vi "poc.test.vi"() -> ()   [LabVIEW 2020]
uses:
  <vilib>/Platform/TimedLoop/XDataNode/timing_clust.ctl
  <vilib>/Platform/TimedLoop/XDataNode/nitl_modes.ctl
  <vilib>/Platform/TimedLoop/XDataNode/wakeup.ctl
  axi_2_eth_raw.ctl
  <vilib>/rvi/DataTransferAndStorage/Container/Common/niFpgaContainerGetUniqueNameForEmu.vi
  <vilib>/rvi/DataTransferAndStorage/Container/Common/niFpgaContainerSetEmuInfo.vi
  <vilib>/rvi/eio/common/nirviEmuReportErrorAndStop.vi
  <vilib>/rvi/Emulation/niFpgaSctlEmulationGetInTimedLoop.vi
  <vilib>/rvi/Emulation/niFpgaEmulationReportErrorSimple.vi
  <vilib>/rvi/Emulation/niFpgaGetClockAttributes.vi
  <vilib>/rvi/Emulation/niFpgaCriticalErrorInLSC.vi
  <vilib>/rvi/DataTransferAndStorage/Container/Common/niFpgaContainerExecOnDevCompGetState.vi
  <vilib>/rvi/Emulation/niFpgaEmulationIsFPGAContextNoSignature.vi
  <vilib>/rvi/errors/niFpgaSetErrorForExecOnDevCompSimple.vi
  <vilib>/rvi/FIFO/Fifo_Resource/nirvififoEmulationSetSize.vi
  <vilib>/rvi/FIFO/Fifo_Resource/nirviFifoEmulationQueueMgr.vi
  <instcachedir>/0/nirviFifoEmulationQueueMgr_E5CAEC123FF24DC58D834DCA3CDAA9B5.lvgen/nirviFifoEmulationQueueMgr_E5CAEC123FF24DC58D834DCA3CDAA9B5_018.vi
  <vilib>/rvi/FIFO/Fifo_Resource/nirvififoEmulationDetermineInputValidOut.vi
  <vilib>/rvi/FIFO/Fifo_Resource/nirvififoEmulationCreateLock.vi
  <vilib>/rvi/Emulation/niFpgaProcessEmulError.vi
  <vilib>/rvi/FIFO/Fifo_Resource/nirvififoEmulationObtainLock.vi
  <vilib>/rvi/FIFO/Fifo_Resource/nirvififoEmulationReleaseLock.vi
  <vilib>/rvi/occurrence/nirviWaitOnOccurrenceBase.vi
  <vilib>/rvi/errors/nirviReportUnexpectedCaseInternalError.vi
  <vilib>/rvi/errors/nirviReportUnexpectedCaseInternalError (U32).vi
  <vilib>/Utility/error.llb/Clear Errors.vi
  <vilib>/rvi/interface/RandomDataEmulation/niFpgaRandomDataHandleErrors.vi
  <instcachedir>/0/nirviFifoEmulationQueueMgr_E5CAEC123FF24DC58D834DCA3CDAA9B5.lvgen/nirviFifoEmulationQueueMgr_E5CAEC123FF24DC58D834DCA3CDAA9B5_020.vi
  <vilib>/rvi/interface/RandomDataEmulation/nirviRandomDataMultiElementFPGAFIFO.vi
  <instcachedir>/0/nirviRandomDataMultiElementFPGAFIFO_3E9965BA1FAD4E7B8DABA31768A09B1F.lvgen/nirviRandomDataMultiElementFPGAFIFO_3E9965BA1FAD4E7B8DABA31768A09B1F_001.vi
  <instcachedir>/0/nirviFifoEmulationQueueMgr_E5CAEC123FF24DC58D834DCA3CDAA9B5.lvgen/nirviFifoEmulationQueueMgr_E5CAEC123FF24DC58D834DCA3CDAA9B5_017.vi
  <vilib>/rvi/Memory/Memory_Emulation/niFpgaMemoryEmulationCacheClearOnFirstRun.vi
  <vilib>/rvi/Memory/Memory_Emulation/nirvimemoryEmulationManagerCache_MakeExclusive.vi
  <vilib>/rvi/Memory/Memory_Emulation/niFpgaMemoryEmulationValidateCache.vi
  <vilib>/rvi/Memory/Memory_Emulation/nirvimemoryEmulationManagerCache_InsertValue.vi
  <vilib>/rvi/Memory/Memory_Emulation/nirvimemoryEmulationManagerCache_ReleaseExclusive.vi
  <vilib>/rvi/Memory/Memory_Emulation/nirvimemoryEmulationManagerCache_GetValue.vi
  <vilib>/rvi/Memory/Memory_Emulation/nirvimemoryEmulationManagerCache_SetValue.vi
  <vilib>/rvi/Emulation/niFpgaSctlEmulationResourceMgr.vi
  <vilib>/Platform/TimedLoop/XDataNode/XDataNode.xnode
  <vilib>/rvi/LocalResourceManager/LocalResourceManager.xnode
  <vilib>/rvi/DataTransferAndStorage/Container/XNode/niFpgaContainer.xnode
  <vilib>/rvi/FIFO/Fifo_Resource/niFpgaFifoEmulationRefIn.vi
  <vilib>/rvi/FIFO/Fifo_Resource/nirvififoEmulationRead.vi
  <vilib>/rvi/interface/RandomDataEmulation/nirviRandomDataFpgaMultiElementTemplate.vi
  <vilib>/rvi/Memory/Memory_Emulation/niFpgaMemoryEmulationRefIn.vi
  <vilib>/Platform/TimedLoop/XDataNode/XDNodeRunTimeDep.lvlib
  submodules/Market.Data.Common/fpga/fpganow.common.fpga.lvlib
panel:
  in  "ip.Reset":bool
  out "i":u16
  out "Data":T1
  out "Numeric":i32
  in  "Reset":bool
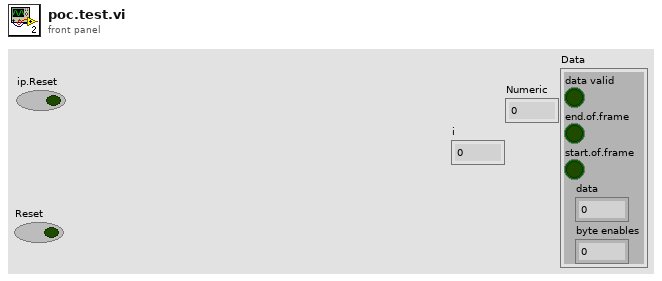
[diagram p1: front panel]
types:
  T1 = cluster{"data valid":bool, "end.of.frame":bool, "start.of.frame":bool, "data":u64, "byte enables":u8}
  T2 = typedef "XDNodeRunTimeDep.lvlib/timing_clust.ctl" = cluster{"Expected End [f-1]":u64, "Actual End [f-1]":u64, "Finished Late? [f-1]":bool, "Expected End [i-1]":u64, "Actual End [i-1]":u64, "Finished Late? [i-1]":bool, "Expected Start [i]":u64, "Actual Start [i]":u64, "Expected Start [f]":u64, "Actual Start [f]":u64, "Source Name":string, "Structure Name":string, "Period":i64, "Deadline":i64, "Offset":i64, "Start":i64, "Priority":i32, "Timeout":i32, "Mode":T3, "Wakeup Reason":T4, "Error":errorcluster, "Source Type":string, "Secondary Source Type":string, "Global End Time":u64, "Global Start Time":u64, "Frame Duration":u64, "Iteration Duration":u64, "Assigned CPU":i32, "I/O Scan Engine Mode":u32}
  T3 = typedef "XDNodeRunTimeDep.lvlib/nitl_modes.ctl" = enum32{"No Change", "Process missed periods, maintain original phase", "Discard missed periods, maintain original phase", "Process missed periods, ignore original phase", "Discard missed periods, ignore original phase"}
  T4 = typedef "XDNodeRunTimeDep.lvlib/wakeup.ctl" = enum32{"Normal", "Aborted", "Asynchronous wakeup", "Timing source error", "Timed loop error", "Timeout"}
  T5 = typedef "axi_2_eth_raw.ctl" = cluster{"data valid":bool, "end.of.frame":bool, "start.of.frame":bool, "data":u64, "byte enables":u8}
  T6 = cluster{"type":enum8{"Time", "AddOrder", "OrderExecuted", "OrderExecutedAtPrice", "ReduceSize", "ModifyOrder", "DeleteOrder", "Get.Everything", "Get.All.Orders", "Get.Top"}, "side":u8, "orderId ":u64, "quantity":u32, "symbol":u64, "price":u64, "executed.qty":u32, "canceled.qty":u32, "remaining.qty":u32, "seconds":u64, "nanoseconds":u64, "Add":bool, "Edit":bool, "Remove":bool, "seq no":u32, "recv.time":u64, "parse.time":u64}
  T7 = enum8{"Time", "AddOrder", "OrderExecuted", "OrderExecutedAtPrice", "ReduceSize", "ModifyOrder", "DeleteOrder", "Get.Everything", "Get.All.Orders", "Get.Top"}
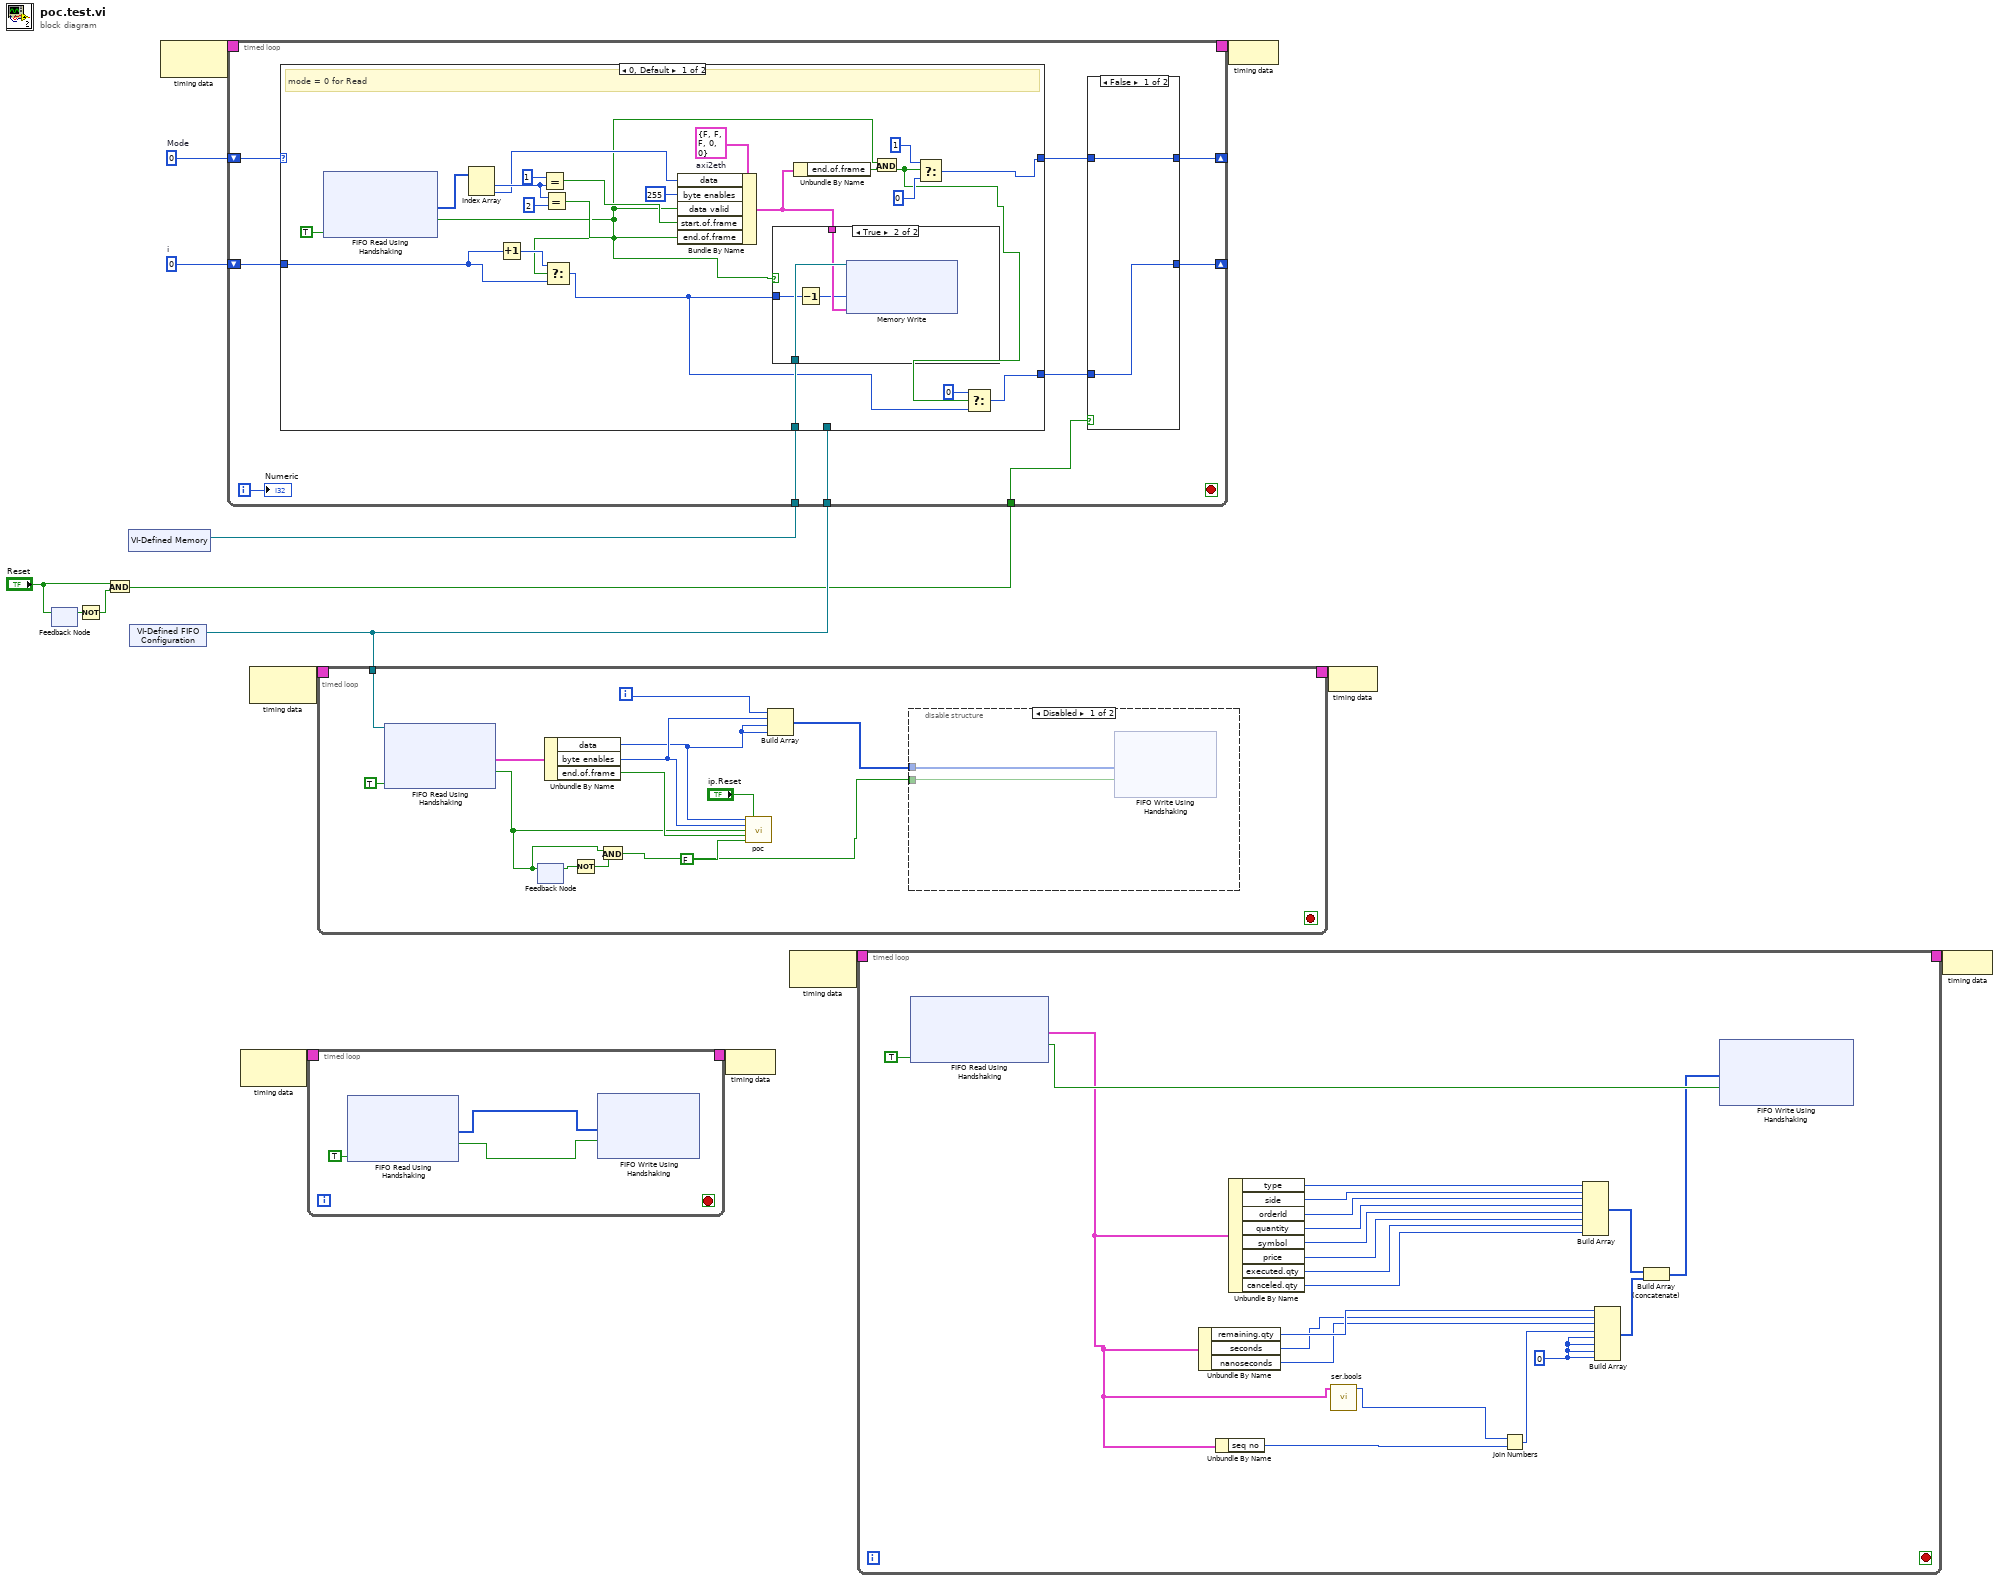
[diagram p0: block diagram]
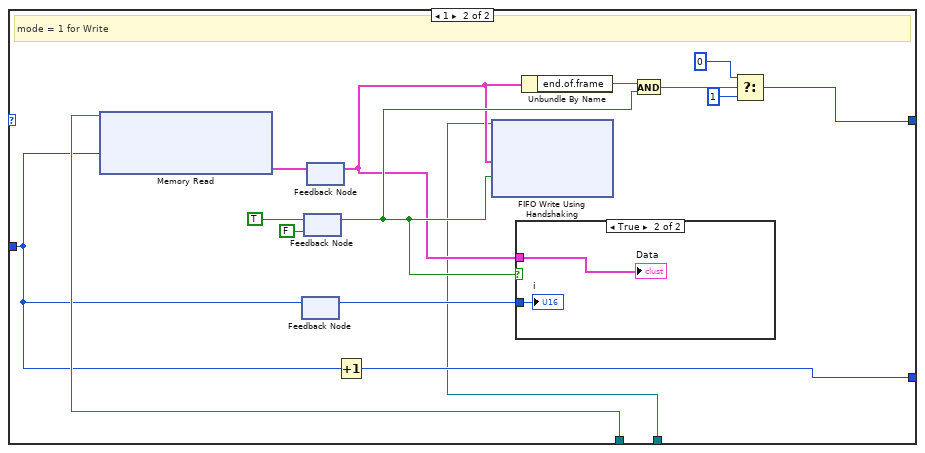
[diagram p4: hidden frame]
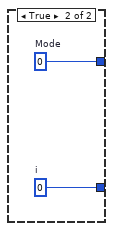
[diagram p6: hidden frame]
diagram:
  w6 = u16 0  # i
  w7 = u8 0  # Mode
  n1 = feedback-in #1("Reset") -> ()
  n2 = feedback #1() -> (w11:bool)  [unwired: 1 in]
  n3 = Not(x=w11) -> (.not. x?=w10:bool)
  n4 = And(x="Reset", y=w10) -> (x .and. y?=w8:bool)
  n5 = xnode "VI-Defined Memory"() -> ("Memory Out"=w5:refnum<k21>)
  n6 = xnode "VI-Defined FIFO Configuration"() -> ("FIFO Out"=w12:refnum<k21>)
  n7 = node-c288() -> (w16:T2)  [unwired: 1 in]
  n8 = timed-loop {
    timing: w16 -> [_]
    timing-out: [_] -> w15
    tunnel: w12 -> [w18]
    tunnel: w8 -> [w21]
    shift-right: [w26] -> _
    shift-left: w7 -> [w25]
    shift-right: [w24] -> _
    shift-left: w6 -> [w23]
    tunnel: w5 -> [w22]
    i -> [w17]
    stop <- _ stop-if-true
    n9 = case shown="0, Default" w25 {
      tunnel: w23 -> [w38 w56]
      tunnel: w22 -> [w37 w68]
      tunnel: [w30 w62] -> w20
      tunnel: [w32 w65] -> w19
      tunnel: w18 -> [_ w54]
      frame 0, Default {
        w49 = T5 {"data valid"=FALSE, "end.of.frame"=FALSE, "start.of.frame"=FALSE, "data"=0, "byte enables"=0}  # axi2eth
        # "mode = 0 for Read"
        n10 = xnode "FIFO Read Using Handshaking"("Ready for Output"=TRUE) -> ("Element"=w48:u64[], "Output Valid"=w31:bool)  [unwired: 1 in, 1 out]
        n11 = Index Array(array=w48) -> (element #1=w47:u64, element #2=w41:u64)  [unwired: 2 in]
        n12 = Increment(x=w38) -> (x+1=w39:u16)
        n13 = Equal?(x=u64 1, y=w47) -> (x = y?=w43:bool)
        n14 = Equal?(x=w47, y=u64 2) -> (x = y?=w44:bool)
        n15 = Select(t=w39, s=w31, f=w38) -> (s? t:f=w29:u16)
        n16 = Bundle By Name(cluster=w49, "data"=w41, "byte enables"=u8 255 ("number"), "data valid"=w31, "start.of.frame"=w43, "end.of.frame"=w44) -> (w36:T5)
        n17 = case shown="True" w31 {
          tunnel: w37 -> [_ w53]
          tunnel: w36 -> [_ w52]
          tunnel: w29 -> [_ w51]
          frame False {
          }
          frame True {
            n18 = Decrement(x=w51) -> (x-1=w50:u16)
            n19 = xnode "Memory Write"("Address"=w50, "Data"=w52, "Memory In"=w53) -> ()  [unwired: 1 out]
          }
        }
        n20 = Unbundle By Name(w36) -> ("end.of.frame"=w35:bool)
        n21 = And(x=w31, y=w35) -> (x .and. y?=w28:bool)
        n22 = Select(t=u8 1, s=w28, f=u8 0 ("t")) -> (s? t:f=w32:u8)
        n23 = Select(t=u16 0, s=w28, f=w29) -> (s? t:f=w30:u16)
      }
      frame 1 {
        # "mode = 1 for Write"
        n24 = xnode "Memory Read"("Address"=w56, "Memory In"=w68) -> ("Data"=w67:T1)  [unwired: 1 out]
        n25 = feedback-in #2(w56) -> ()
        n26 = feedback #2() -> (w55:u16)  [unwired: 1 in]
        n27 = feedback-in #3(TRUE ("Input Valid")) -> ()
        n28 = feedback #3(FALSE ("Input Valid")) -> (w58:bool)
        n29 = feedback-in #4(w67) -> ()
        n30 = feedback #4() -> (w57:T1)  [unwired: 1 in]
        n31 = Increment(x=w56) -> (x+1=w62:u16)
        n32 = xnode "FIFO Write Using Handshaking"("Element"=w57, "Input Valid"=w58, "FIFO In"=w54) -> ()  [unwired: 2 out]
        n33 = case shown="True" w58 {
          tunnel: w57 -> [_ w70]
          tunnel: w55 -> [_ w69]
          frame False {
          }
          frame True {
            "Data" <- w70
            "i" <- w69
          }
        }
        n34 = Unbundle By Name(w57) -> ("end.of.frame"=w66:bool)
        n35 = And(x=w66, y=w58) -> (x .and. y?=w59:bool)
        n36 = Select(t=u8 0 ("f"), s=w59, f=u8 1) -> (s? t:f=w65:u8)
      }
    }
    n37 = case shown="False" w21 {
      tunnel: [w71 w74] -> w26
      tunnel: [w72 w73] -> w24
      tunnel: w20 -> [w72 _]
      tunnel: w19 -> [w71 _]
      frame False {
      }
      frame True {
        w73 = u16 0  # i
        w74 = u8 0  # Mode
      }
    }
    "Numeric" <- w17
  }
  n38 = node-c288() -> (w2:T2)  [unwired: 1 in]
  n39 = node-c288() -> (w14:T2)  [unwired: 1 in]
  n40 = timed-loop {
    timing: w2 -> [_]
    timing-out: [_] -> w1
    stop <- _ stop-if-true
    n41 = xnode "FIFO Read Using Handshaking"("Ready for Output"=TRUE) -> ("Element"=w77:u64[], "Output Valid"=w78:bool)  [unwired: 1 in, 1 out]
    n42 = xnode "FIFO Write Using Handshaking"("Element"=w77, "Input Valid"=w78) -> ()  [unwired: 1 in, 2 out]
  }
  n43 = timed-loop {
    timing: w14 -> [_]
    timing-out: [_] -> w13
    tunnel: w12 -> [w95]
    i -> [w85]
    stop <- _ stop-if-true
    n44 = xnode "FIFO Read Using Handshaking"("Ready for Output"=TRUE, "FIFO In"=w95) -> ("Element"=w86:T1, "Output Valid"=w84:bool)  [unwired: 1 out]
    n45 = feedback-in #5(w84) -> ()
    n46 = feedback #5() -> (w90:bool)  [unwired: 1 in]
    n47 = Unbundle By Name(w86) -> ("data"=w82:u64, "byte enables"=w87:u8, "end.of.frame"=w92:bool)
    n48 = Not(x=w90) -> (.not. x?=w89:bool)
    n49 = And(x=w84, y=w89) -> (x .and. y?=w83:bool)
    n50 = call "poc.vi"("TDATA"=w82, "reset"="ip.Reset", "TKEEP"=w87, "TVALID"=w84, "TLAST"=w92, "TUSER"=FALSE) -> ()  [unwired: 10 in]
    n51 = Build Array(w85, w87, w82, w82) -> (w88:u64[])
    n52 = disable-structure shown="Disabled" {
      disable-tunnel: w83 -> [w97 _]
      disable-tunnel: w88 -> [w96 _]
      frame Disabled {
        n53 = xnode "FIFO Write Using Handshaking"("Element"=w96, "Input Valid"=w97) -> ()  [unwired: 1 in, 2 out]
      }
      frame Enabled {
      }
    }
  }
  n54 = node-c288(w1) -> ()
  n55 = node-c288() -> (w4:T2)  [unwired: 1 in]
  n56 = timed-loop {
    timing: w4 -> [_]
    timing-out: [_] -> w3
    stop <- _ stop-if-true
    w107 = u64 0 ("element")
    n57 = xnode "FIFO Read Using Handshaking"("Ready for Output"=TRUE) -> ("Element"=w100:T6, "Output Valid"=w119:bool)  [unwired: 1 in, 1 out]
    n58 = Unbundle By Name(w100) -> ("remaining.qty"=w108:u32, "seconds"=w105:u64, "nanoseconds"=w106:u64)
    n59 = Unbundle By Name(w100) -> ("seq no"=w103:u32)
    n60 = Unbundle By Name(w100) -> ("type"=w118:T7, "side"=w117:u8, "orderId"=w116:u64, "quantity"=w115:u32, "symbol"=w114:u64, "price"=w113:u64, "executed.qty"=w112:u32, "canceled.qty"=w111:u32)
    n61 = call "ser.bools.vi"("orderbook.command"=w100) -> ("Numeric"=w101:u32)  [unwired: 10 in]
    n62 = Join Numbers(hi=w101, lo=w103) -> ((hi.lo)=w104:u64)
    n63 = Build Array(w118, w117, w116, w115, w114, w113, w112, w111) -> (w110:u64[])
    n64 = Build Array(w108, w105, w106, w104, w107, w107, w107, w107) -> (w109:u64[])
    n65 = Build Array (concatenate)(w110, w109) -> (w102:u64[])
    n66 = xnode "FIFO Write Using Handshaking"("Element"=w102, "Input Valid"=w119) -> ()  [unwired: 1 in, 2 out]
  }
  n67 = node-c288(w15) -> ()
  n68 = node-c288(w13) -> ()
  n69 = node-c288(w3) -> ()
